vi "PXI_Host_U64_Read_OldMethod_Benchmark.vi"() -> ()   [LabVIEW 2018]
uses:
  <vilib>/Platform/TimedLoop/XDataNode/timing_clust.ctl
  <vilib>/Platform/TimedLoop/XDataNode/nitl_modes.ctl
  <vilib>/Platform/TimedLoop/XDataNode/wakeup.ctl
  <vilib>/addons/FPGA Advanced Session Resources/LVFPGA Adv Session Resources/OpenByNameSubVI.vi
  <vilib>/rvi/interface/common/dynamic/niFpgaEscapeDelimiterAndNull.vi
  <vilib>/Utility/error.llb/Error Cluster From Error Code.vi
  <vilib>/rvi/errors/niLvFpgaAdjustHostInterfaceError.vi
  <vilib>/FPGAPlugInAG/Dynamic/niLvFpga_Close_Dynamic.vi
  <vilib>/addons/FPGA Advanced Session Resources/LVFPGA Adv Session Resources/OpenByName.xnode
  <vilib>/platform/TimedLoop/XDataNode/XDataNode.xnode
  <vilib>/rvi/interface/nirviReadWriteControl/nirviReadWriteControl.xnode
  <vilib>/rvi/interface/nirviCloseFPGA/nirviCloseFPGA.xnode
  NiFpgaLv.dll
  <vilib>/rvi/interface/Simulation/niFpgaSimulationCallBeginRW.vi
  <vilib>/Platform/TimedLoop/XDataNode/XDNodeRunTimeDep.lvlib
  <vilib>/addons/FPGA Advanced Session Resources/LVFPGA Adv Session Resources/LVFPGAAdvSessionResources.lvlib
panel:
  out "Standard Dev":dbl
  out "Execution time (s)":dbl
  out "Maximum(s)":dbl
  out "Waveform Graph":dbl[](graph)
  out "Value out":u64
  out "error out":errorcluster
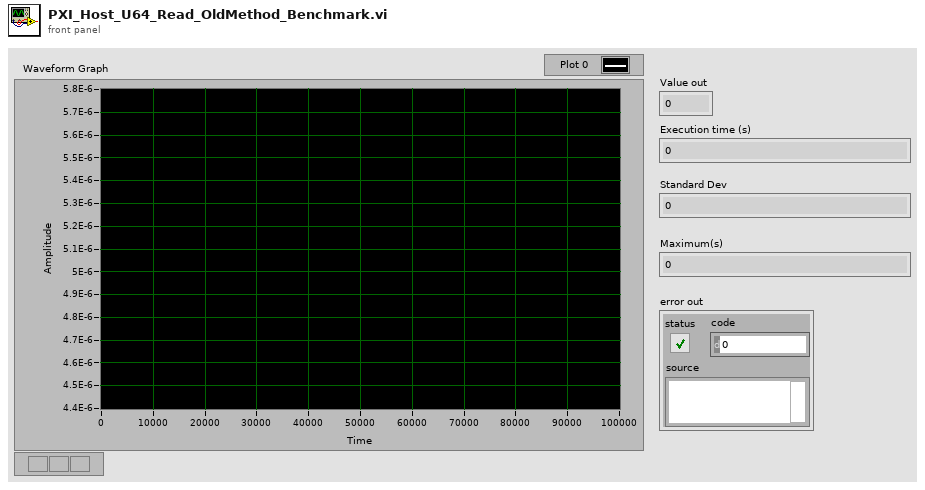
[diagram p1: front panel]
types:
  T1 = typedef "XDNodeRunTimeDep.lvlib/timing_clust.ctl" = cluster{"Expected End [f-1]":u64, "Actual End [f-1]":u64, "Finished Late? [f-1]":bool, "Expected End [i-1]":u64, "Actual End [i-1]":u64, "Finished Late? [i-1]":bool, "Expected Start [i]":u64, "Actual Start [i]":u64, "Expected Start [f]":u64, "Actual Start [f]":u64, "Source Name":string, "Structure Name":string, "Period":i64, "Deadline":i64, "Offset":i64, "Start":i64, "Priority":i32, "Timeout":i32, "Mode":T2, "Wakeup Reason":T3, "Error":errorcluster, "Source Type":string, "Secondary Source Type":string, "Global End Time":u64, "Global Start Time":u64, "Frame Duration":u64, "Iteration Duration":u64, "Assigned CPU":i32, "I/O Scan Engine Mode":u32}
  T2 = typedef "XDNodeRunTimeDep.lvlib/nitl_modes.ctl" = enum32{"No Change", "Process missed periods, maintain original phase", "Discard missed periods, maintain original phase", "Process missed periods, ignore original phase", "Discard missed periods, ignore original phase"}
  T3 = typedef "XDNodeRunTimeDep.lvlib/wakeup.ctl" = enum32{"Normal", "Aborted", "Asynchronous wakeup", "Timing source error", "Timed loop error", "Timeout"}
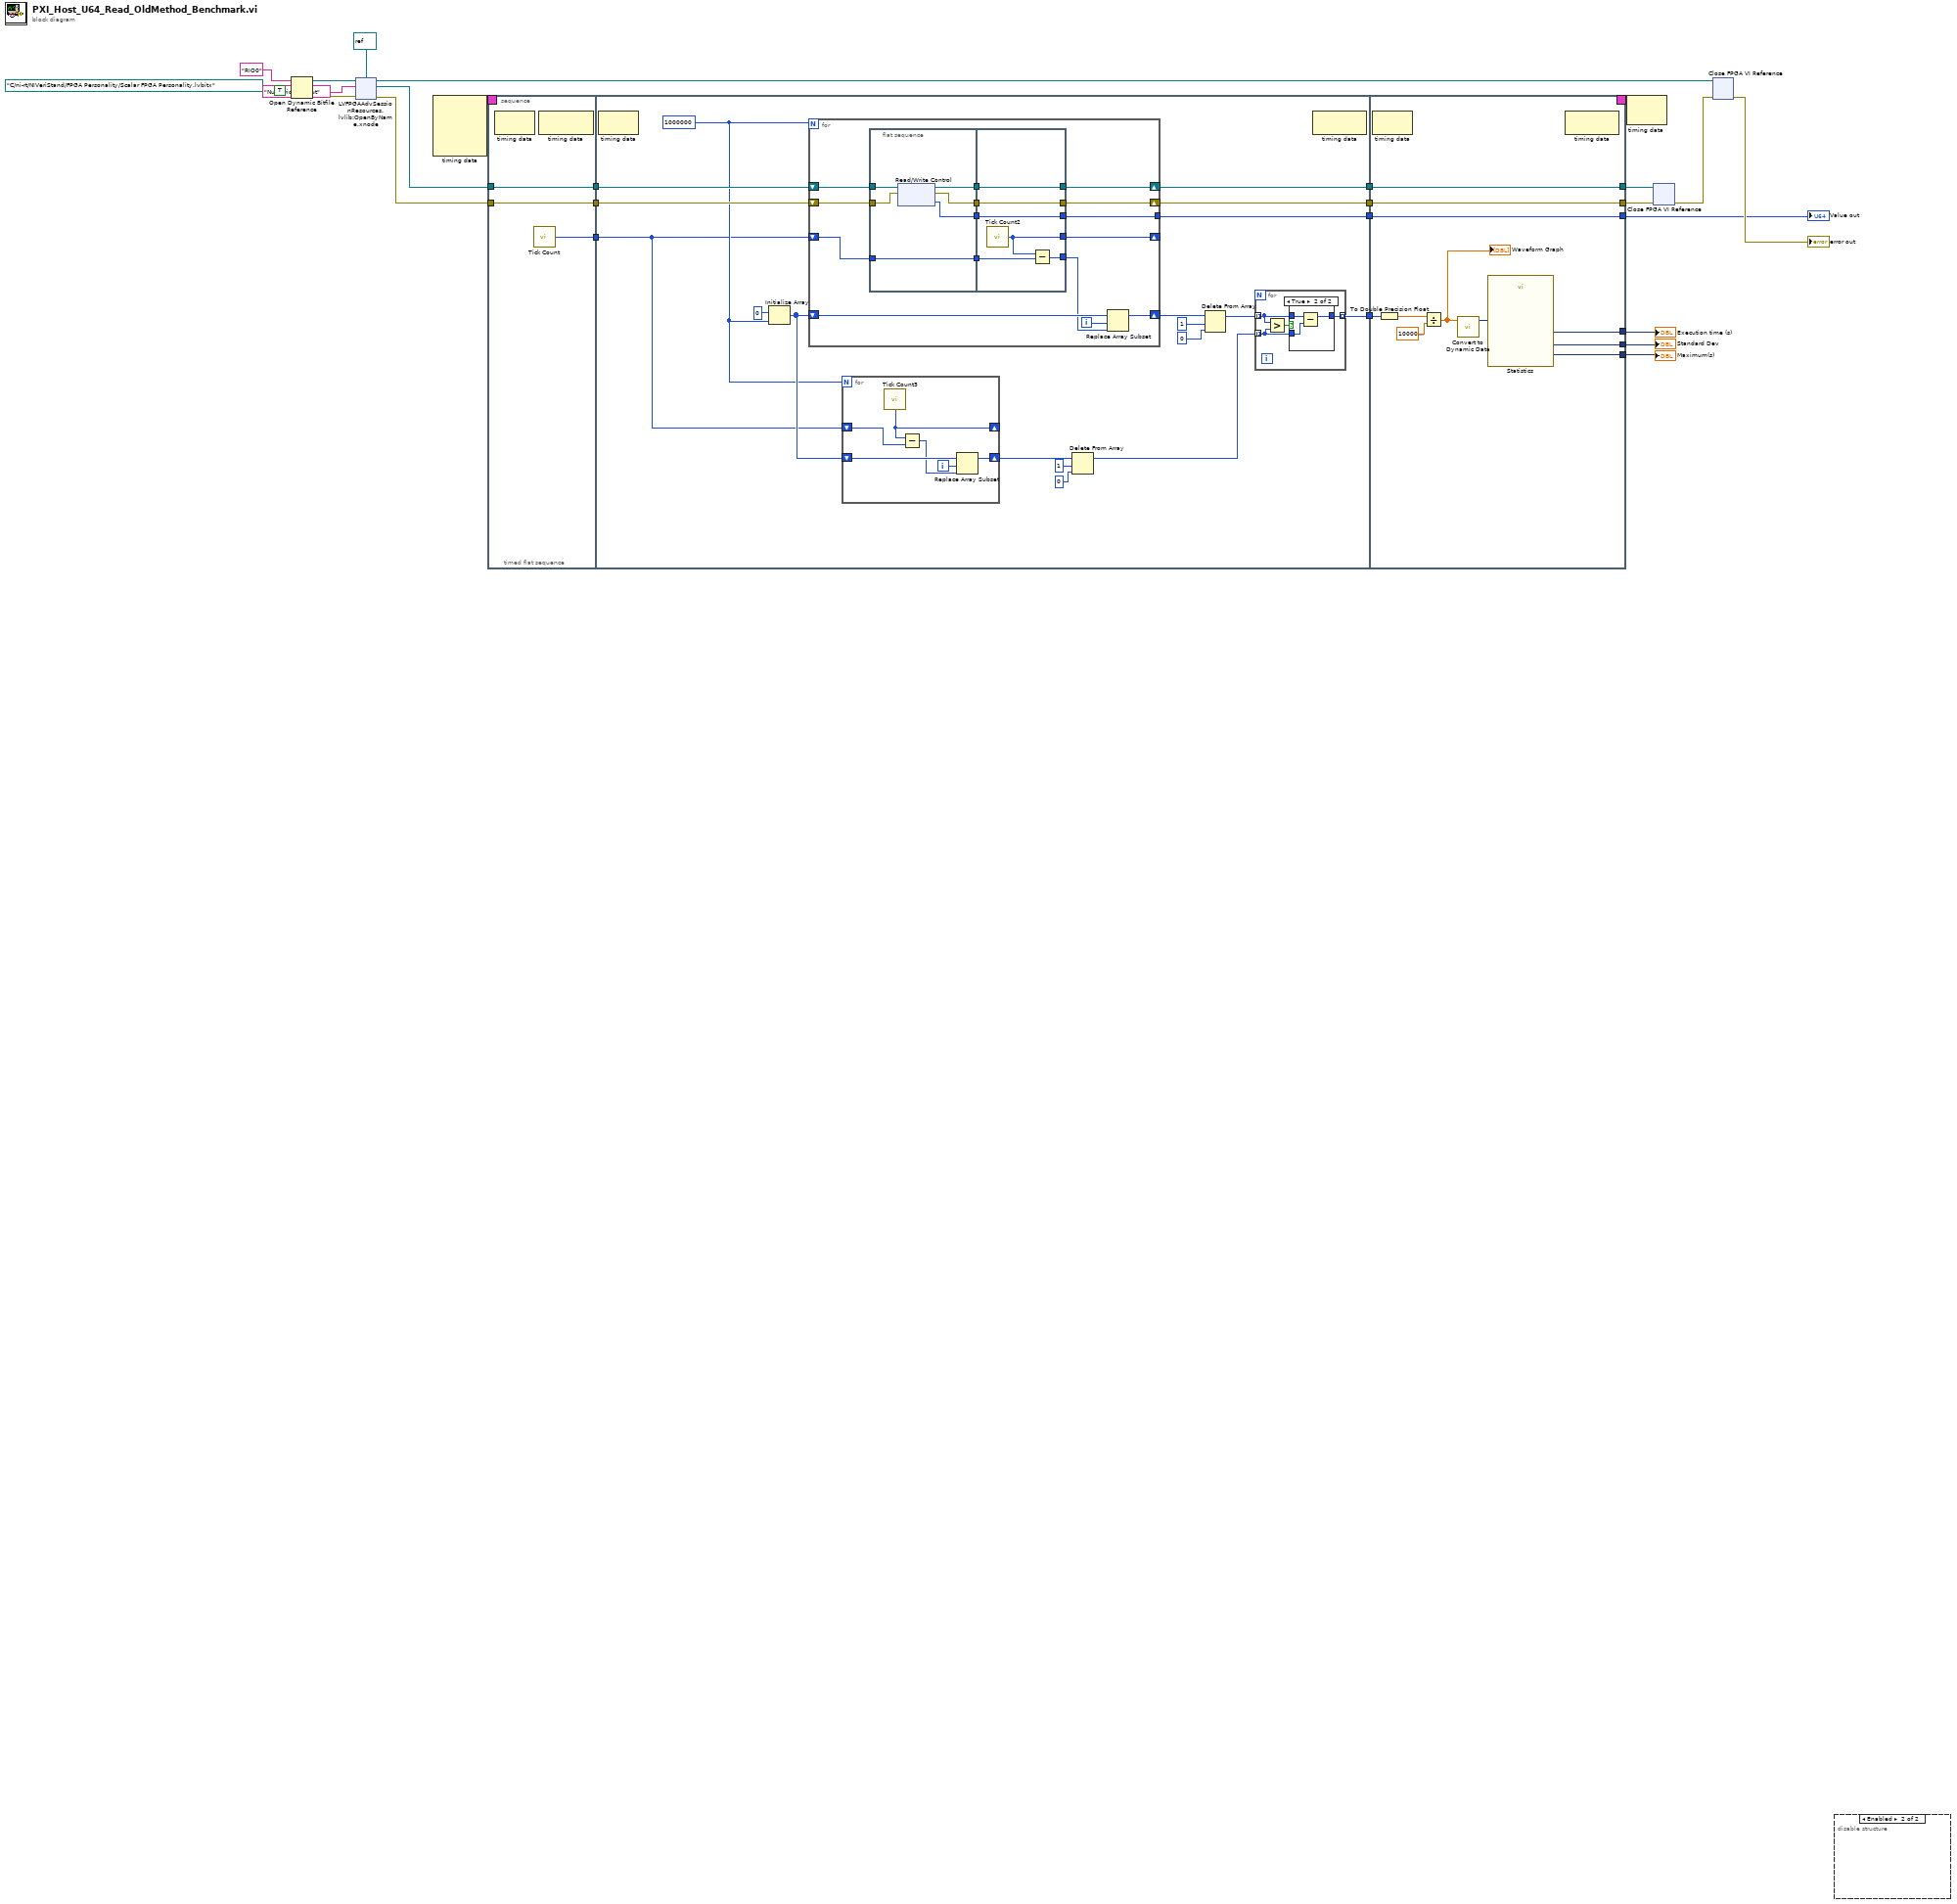
[diagram p0: block diagram]
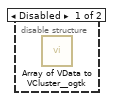
[diagram p3: hidden frame]
diagram:
  n1 = Open Dynamic Bitfile Reference(0:"RIO0" ("Device address"), 1:path "C:/ni-rt/NIVeriStand/FPGA Personality/Scalar FPGA Personality.lvbitx" ("Bitfile path"), 2:TRUE ("Run When Loaded")) -> (5:w16:refnum<k20>, 8:w14:errorcluster)  [unwired: 2 in]
  n2 = xnode "LVFPGAAdvSessionResources.lvlib:OpenByName.xnode"("FPGA VI Reference in"=w16, "Resource name in"="Numeric U64 out", "Single resource reference type in"=refnum<k20> refnum ("Type"), "Error in"=w14) -> ("Single resource reference out"=w12:refnum<k20>, "Error out"=w13:errorcluster, "FPGA VI Reference out"=w8:refnum<k20>)
  n3 = node-c288() -> (w5:T1)  [unwired: 4 in]
  n4 = timed-sequence {
    timing: w5 -> [_]
    timing-out: [_] -> w4
    tunnel: [w35] -> w17
    tunnel: w13 -> [w34]
    tunnel: w12 -> [w33]
    tunnel: [w32] -> w10
    tunnel: [w31] -> w6
    tunnel: [w23] -> w3
    tunnel: [w22] -> w2
    tunnel: [w21] -> w1
    n5 = timed-flat-sequence {
      tunnel: w33 -> [w37]
      tunnel: w34 -> [w38]
      tunnel: [w38] -> w30
      tunnel: [w37] -> w29
      tunnel: [w36] -> w28
      tunnel: w30 -> [w57]
      tunnel: w29 -> [w56]
      tunnel: w28 -> [w44]
      tunnel: [w58] -> w27
      tunnel: [w55] -> w26
      tunnel: [w54] -> w25
      tunnel: [w41] -> w24
      tunnel: [w110] -> w31
      tunnel: [w111] -> w32
      tunnel: [w112] -> w35
      tunnel: w27 -> [w112]
      tunnel: w26 -> [w111]
      tunnel: w25 -> [w110]
      tunnel: w24 -> [w105]
      tunnel: [w104] -> w23
      tunnel: [w103] -> w22
      tunnel: [w102] -> w21
      frame #0 {
        n6 = node-c288() -> ()  [unwired: 1 in, 1 out]
        n7 = call "Tick Count"() -> ("Tick Count(Ticks)"=w36:u32)
        n8 = node-c288() -> ()  [unwired: 1 in, 1 out]
      }
      frame #1 {
        w45 = 1000000
        n9 = node-c288() -> ()  [unwired: 1 in, 1 out]
        n10 = Initialize Array(u32 0 ("Tick Count(uSec)"), w45) -> (w46:u32[])
        n11 = for {
          N: w45 -> [_]
          tunnel: [w82] -> w54
          shift-right: [w86] -> w58
          shift-left: w57 -> [w85]
          shift-right: [w83] -> w55
          shift-left: w56 -> [w84]
          shift-right: [w79] -> _
          shift-left: w44 -> [w81]
          shift-right: [w77] -> w42
          shift-left: w46 -> [w78]
          i -> [w75]
          n12 = flat-sequence {
            tunnel: [w93] -> w89
            tunnel: [w92] -> w88
            tunnel: [w91] -> w87
            tunnel: w84 -> [w95]
            tunnel: w85 -> [w94]
            tunnel: w81 -> [w90]
            tunnel: [w90] -> w80
            tunnel: w89 -> [w101]
            tunnel: [w101] -> w86
            tunnel: [w100] -> w82
            tunnel: w88 -> [w100]
            tunnel: w87 -> [w99]
            tunnel: [w99] -> w83
            tunnel: w80 -> [w98]
            tunnel: [w97] -> w79
            tunnel: [w96] -> w76
            frame #0 {
              n13 = xnode "Read/Write Control"("FPGA VI Reference In"=w95, "error in"=w94) -> ("FPGA VI Reference Out"=w91:refnum<k20>, "error out"=w93:errorcluster, "Value"=w92:u64)
            }
            frame #1 {
              n14 = call "Tick Count2"() -> ("Tick Count(Ticks)"=w97:u32)
              n15 = Subtract(x=w97, y=w98) -> (x-y=w96:u32)
            }
          }
          n16 = Replace Array Subset(array=w78, new element=w76, index=w75) -> (w77:u32[])
        }
        n17 = for {
          N: w45 -> [_]
          shift-right: [w69] -> w48
          shift-left: w46 -> [w72]
          shift-right: [w74] -> _
          shift-left: w44 -> [w73]
          i -> [w70]
          n18 = call "Tick Count3"() -> ("Tick Count(Ticks)"=w74:u32)
          n19 = Subtract(x=w74, y=w73) -> (x-y=w71:u32)
          n20 = Replace Array Subset(array=w72, new element=w71, index=w70) -> (w69:u32[])
        }
        n21 = Delete From Array(array=w48, length=1, index=0) -> (array with subset deleted=w43:u32[])  [unwired: 1 out]
        n22 = Delete From Array(array=w42, length=1, index=0) -> (array with subset deleted=w47:u32[])  [unwired: 1 out]
        n23 = for {
          tunnel: [w64] -> w41 mode=indexing
          tunnel: w47 -> [w63] mode=indexing
          tunnel: w43 -> [w62] mode=indexing
          n24 = Greater?(x=w63, y=w62) -> (0:w61:bool)
          n25 = case shown="True" w61 {
            tunnel: w63 -> [w65 w68]
            tunnel: w62 -> [_ w67]
            tunnel: [w65 w66] -> w64
            frame False {
            }
            frame True {
              n26 = Subtract(x=w68, y=w67) -> (x-y=w66:u32)
            }
          }
        }
        n27 = node-c288() -> ()  [unwired: 1 in, 1 out]
      }
      frame #2 {
        n28 = node-c288() -> ()  [unwired: 1 in, 1 out]
        n29 = To Double Precision Float(number=w105) -> (double precision float=w109:dbl[])
        n30 = Divide(x=w109, y=1000000000.0) -> (x/y=w106:dbl[])
        "Waveform Graph" <- w106
        n31 = call "Convert to Dynamic Data"("Array"=w106) -> ("Dynamic Data Type"=w107:dynamicdata)  [unwired: 3 in]
        n32 = call "Statistics"("Signals"=w107) -> ("Standard Dev"=w103:dynamicdata, "Arithmetic Mean"=w104:dynamicdata, "Maximum"=w102:dynamicdata)  [unwired: 23 in, 1 out]
        n33 = node-c288() -> ()  [unwired: 1 in, 1 out]
      }
    }
  }
  "Value out" <- w6
  "Maximum(s)" <- w1
  "Execution time (s)" <- w3
  "Standard Dev" <- w2
  n34 = node-c288(w4) -> ()  [unwired: 1 out]
  n35 = xnode "Close FPGA VI Reference"("FPGA VI Reference In"=w10, "error in"=w17) -> ("error out"=w9:errorcluster)
  n36 = xnode "Close FPGA VI Reference"("FPGA VI Reference In"=w8, "error in"=w9) -> ("error out"=→"error out":errorcluster)
  n37 = disable-structure shown="Enabled" {
    frame Disabled {
      n38 = call <userlib>:"Array of VData to VCluster__ogtk.vi"() -> ()  [unwired: 10 in, 2 out]
    }
    frame Enabled {
    }
  }
